vi "01-main.vi"() -> ()   [LabVIEW 2015]
panel:
  out "get_bus_statistics":dbl
  out "get_can_channel_count":i32
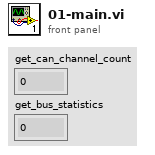
[diagram p1: front panel]
types:
  T1 = cluster{"channel":i32, "extended？":bool, "id":i32, "dlc":i32, "data":string, "ms":i32}
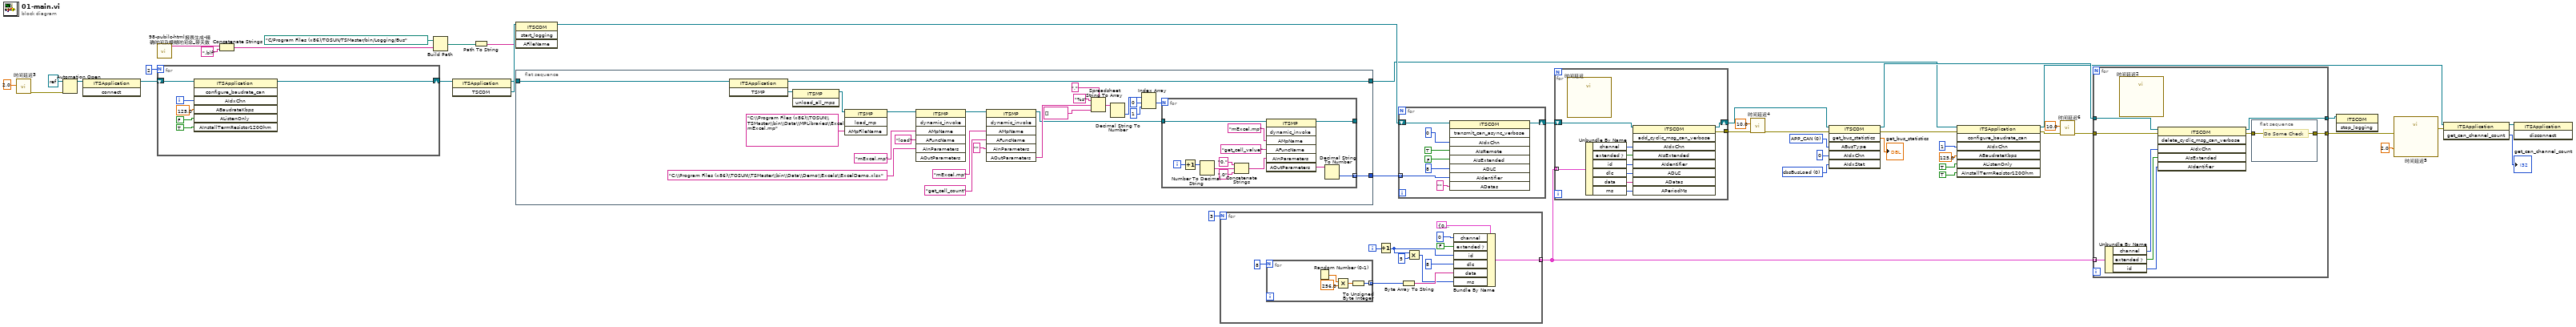
[diagram p0: block diagram]
diagram:
  w21 = 0 items=["cbsBusLoad", "cbsPeakLoad", "cbsFpsStdData", "cbsAllStdData", "cbsFpsExtData", "cbsAllExtData", "cbsFpsStdRemote", "cbsAllStdRemote", "cbsFpsExtRemote", "cbsAllExtRemote", "cbsFpsErrorFrame", "cbsAllErrorFrame"] ("AIdxStat")
  w22 = 0 items=["APP_CAN", "APP_LIN"] ("ABusType")
  n1 = call "时间延迟3"("Delay Time (s)"=2.0) -> ("error out"=w41:errorcluster)  [unwired: 10 in]
  n2 = Automation Open(error in (no error)=w41, Automation Refnum=refnum<k7> refnum ("TSMaster.ITSApplication")) -> (Automation Refnum=w18:refnum<k7>)  [unwired: 2 in, 1 out]
  n3 = invoke on="调用节点" class="ITSApplication" method="connect"(reference=w18) -> (reference out=w17:refnum<k7>)  [unwired: 2 in, 2 out]
  n4 = call "98-pubilc-html报表生成-精确时间及模糊时间命_带天数.vi"() -> ("带年日带毫秒时间"=w30:string)  [unwired: 8 in, 3 out]
  n5 = for {
    N: 2 -> [_]
    shift-right: [w50] -> w5
    shift-left: w17 -> [w51]
    i -> [w46]
    n6 = invoke on="调用节点" class="ITSApplication" method="configure_baudrate_can"(reference=w51, "AIdxChn"=w46, "ABaudrateKbps"=sgl 125.0, "AListenOnly"=FALSE, "AInstallTermResistor120Ohm"=TRUE) -> (reference out=w50:refnum<k7>)  [unwired: 2 in, 6 out]
  }
  n7 = Concatenate Strings(w30, ".blf" ("字符串")) -> (w28:string)
  n8 = Build Path(base path=path "C:/Program Files (x86)/TOSUN/TSMaster/bin/Logging/Bus" ("基路径"), name or relative path=w28) -> (appended path=w27:path)
  n9 = invoke on="调用节点" class="ITSApplication" method="TSCOM"(reference=w5) -> (reference out=w4:refnum<k7>, "TSCOM"=w34:refnum<k7>)  [unwired: 2 in, 1 out]
  n10 = Path To String(path=w27) -> (string=w26:string)
  n11 = invoke on="调用节点" class="ITSCOM" method="start_logging"(reference=w34, "AFileName"=w26) -> (reference out=w6:refnum<k7>)  [unwired: 2 in, 3 out]
  n12 = flat-sequence {
    tunnel: w4 -> [w75]
    tunnel: [w54] -> w2
    tunnel: [w52] -> w1
    frame #0 {
      n13 = invoke on="调用节点" class="ITSApplication" method="TSMP"(reference=w75) -> (reference out=w52:refnum<k7>, "TSMP"=w74:refnum<k7>)  [unwired: 2 in, 1 out]
      n14 = invoke on="调用节点" class="ITSMP" method="unload_all_mps"(reference=w74) -> (reference out=w73:refnum<k7>)  [unwired: 2 in, 2 out]
      n15 = invoke on="调用节点" class="ITSMP" method="load_mp"(reference=w73, "AMpFileName"="C:\\Program Files (x86)\\TOSUN\\TSMaster\\bin\\Data\\MPLibraries\\Excel\\mExcel.mp") -> (reference out=w71:refnum<k7>)  [unwired: 2 in, 3 out]
      n16 = invoke on="调用节点" class="ITSMP" method="dynamic_invoke"(reference=w71, "AMpName"="mExcel.mp", "AFuncName"="load", "AInParameters"="C:\\Program Files (x86)\\TOSUN\\TSMaster\\bin\\Data\\Demo\\Excels\\ExcelDemo.xlsx") -> (reference out=w65:refnum<k7>)  [unwired: 3 in, 6 out]
      n17 = invoke on="调用节点" class="ITSMP" method="dynamic_invoke"(reference=w65, "AMpName"="mExcel.mp", "AFuncName"="get_cell_count", "AInParameters"="") -> (reference out=w55:refnum<k7>, "AOutParameters"=w64:string)  [unwired: 3 in, 5 out]
      n18 = Spreadsheet String To Array(delimiter (Tab)="," ("分隔符(Tab)"), format string="%s" ("格式字符串"), spreadsheet string=w64, array type (2D Dbl)=string[] []) -> (array=w60:string[])
      n19 = Decimal String To Number(string=w60) -> (number=w59:i32[])  [unwired: 2 in, 1 out]
      n20 = Index Array(array=w59, index #1=0 ("索引"), index #2=1 ("索引")) -> (element #1=w56:i32)  [unwired: 1 out]
      n21 = for {
        N: w56 -> [_]
        tunnel: w55 -> [w85]
        tunnel: [w77] -> w54 mode=indexing
        tunnel: [w76] -> _
        i -> [w83]
        n22 = Increment(x=w83) -> (x+1=w82:i32)
        n23 = Number To Decimal String(number=w82) -> (decimal integer string=w81:string)  [unwired: 1 in]
        n24 = Concatenate Strings("0," ("字符串"), w81, ",0" ("字符串")) -> (w79:string)
        n25 = invoke on="调用节点" class="ITSMP" method="dynamic_invoke"(reference=w85, "AMpName"="mExcel.mp", "AFuncName"="get_cell_value", "AInParameters"=w79) -> (reference out=w76:refnum<k7>, "AOutParameters"=w78:string)  [unwired: 3 in, 5 out]
        n26 = Decimal String To Number(string=w78) -> (number=w77:i32)  [unwired: 2 in, 1 out]
      }
    }
  }
  n27 = for {
    N: 3 -> [_]
    tunnel: [w91] -> w43 mode=indexing
    i -> [w99]
    n28 = for {
      N: 8 -> [_]
      tunnel: [w100] -> w93 mode=indexing
      n29 = Random Number (0-1)() -> (number: 0 to 1=w103:dbl)
      n30 = Multiply(x=w103, y=256.0) -> (x*y=w101:dbl)
      n31 = To Unsigned Byte Integer(number=w101) -> (unsigned 8bit integer=w100:u8)
    }
    n32 = Increment(x=w99) -> (x+1=w90:i32)
    n33 = Byte Array To String(unsigned byte array=w93) -> (string=w92:string)
    n34 = Multiply(x=w90, y=5) -> (x*y=w88:i32)
    n35 = Bundle By Name(cluster=T1 {"channel"=0, "extended？"=FALSE, "id"=0, "dlc"=0, "data"="", "ms"=0} ("message"), "channel"=0 ("AIdxChn"), "extended？"=FALSE ("AIsExtended"), "id"=w90, "dlc"=8 ("ADLC"), "data"=w92, "ms"=w88) -> (w91:T1)
  }
  n36 = for {
    shift-right: [w105] -> w3
    shift-left: w6 -> [w111]
    tunnel: w2 -> [w104] mode=indexing
    n37 = invoke on="调用节点" class="ITSCOM" method="transmit_can_async_verbose"(reference=w111, "AIdxChn"=0, "AIsRemote"=TRUE, "AIsExtended"=FALSE, "ADLC"=8, "AIdentifier"=w104, "ADatas"="") -> (reference out=w105:refnum<k7>)  [unwired: 2 in, 8 out]
  }
  n38 = for {
    shift-right: [w120] -> w25
    shift-left: w3 -> [w121]
    tunnel: w43 -> [w119] mode=indexing
    tunnel: [w112] -> w39
    n39 = call "时间延迟"() -> ()  [unwired: 11 in, 1 out]
    n40 = Unbundle By Name(w119) -> ("channel"=w118:i32, "extended？"=w117:bool, "id"=w116:i32, "dlc"=w115:i32, "data"=w114:string, "ms"=w113:i32)
    n41 = invoke on="调用节点" class="ITSCOM" method="add_cyclic_msg_can_verbose"(reference=w121, "AIdxChn"=w118, "AIsExtended"=w117, "AIdentifier"=w116, "ADLC"=w115, "ADatas"=w114, "APeriodMs"=w113) -> (reference out=w120:refnum<k7>, error out=w112:errorcluster)  [unwired: 2 in, 7 out]
  }
  n42 = call "时间延迟4"("error in (no error)"=w39, "Delay Time (s)"=10.0) -> ("error out"=w23:errorcluster)  [unwired: 9 in]
  n43 = invoke on="调用节点" class="ITSCOM" method="get_bus_statistics"(reference=w25, error in=w23, "ABusType"=w22, "AIdxChn"=0, "AIdxStat"=w21) -> (reference out=w24:refnum<k7>, error out=w11:errorcluster, "get_bus_statistics"=→"get_bus_statistics":dbl)  [unwired: 1 in, 3 out]
  n44 = invoke on="调用节点" class="ITSApplication" method="configure_baudrate_can"(reference=w1, error in=w11, "AIdxChn"=1, "ABaudrateKbps"=sgl 125.0, "AListenOnly"=TRUE, "AInstallTermResistor120Ohm"=TRUE) -> (reference out=w12:refnum<k7>, error out=w8:errorcluster)  [unwired: 1 in, 5 out]
  n45 = call "时间延迟6"("error in (no error)"=w8, "Delay Time (s)"=10.0) -> ("error out"=w7:errorcluster)  [unwired: 9 in]
  n46 = for {
    tunnel: w24 -> [w130]
    tunnel: w43 -> [w129] mode=indexing
    tunnel: w7 -> [w124]
    tunnel: [w123] -> w38
    tunnel: [w122] -> w33
    n47 = Unbundle By Name(w129) -> ("channel"=w128:i32, "extended？"=w127:bool, "id"=w126:i32)
    n48 = call "时间延迟2"() -> ()  [unwired: 11 in, 1 out]
    n49 = invoke on="调用节点" class="ITSCOM" method="delete_cyclic_msg_can_verbose"(reference=w130, error in=w124, "AIdxChn"=w128, "AIsExtended"=w127, "AIdentifier"=w126) -> (reference out=w122:refnum<k7>, error out=w125:errorcluster)  [unwired: 1 in, 4 out]
    n50 = flat-sequence {
      tunnel: w125 -> [w131]
      tunnel: [w131] -> w123
      frame #0 {
        # "Do Some Check"
      }
    }
  }
  n51 = invoke on="调用节点" class="ITSCOM" method="stop_logging"(reference=w33) -> ()  [unwired: 2 in, 3 out]
  n52 = call "时间延迟5"("error in (no error)"=w38, "Delay Time (s)"=2.0) -> ("error out"=w37:errorcluster)  [unwired: 9 in]
  n53 = invoke on="调用节点" class="ITSApplication" method="get_can_channel_count"(reference=w12, error in=w37) -> (reference out=w32:refnum<k7>, "get_can_channel_count"=→"get_can_channel_count":i32)  [unwired: 1 in, 1 out]
  n54 = invoke on="调用节点" class="ITSApplication" method="disconnect"(reference=w32) -> ()  [unwired: 2 in, 3 out]
